vi "GetMetadataCluster.vi"(7 "Message":refnum<class "Message.lvclass">) -> (3 "MetadataCluster":T1 {"AbsoluteTime" format="%<%x %.3X>T"})   [LabVIEW 2020, in "jettl.lvlib" / "Message.lvclass"]
uses:
  Message.lvclass
  LifecycleEnum.ctl
  jettl.lvlib
  TellOriginEnum.ctl
  MetadataCluster.ctl
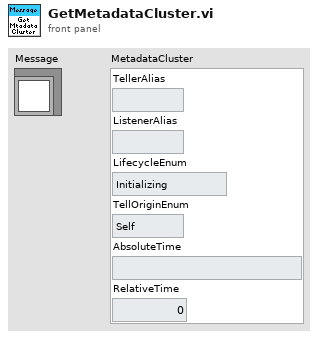
[diagram p1: front panel]
types:
  T1 = typedef "jettl.lvlib/MetadataCluster.ctl" = cluster{"TellerAlias":string, "ListenerAlias":string, "LifecycleEnum":T2, "TellOriginEnum":T3, "AbsoluteTime":timestamp, "RelativeTime":dbl}
  T2 = typedef "jettl.lvlib/LifecycleEnum.ctl" = enum16{"Initializing", "SettingUp", "Starting", "Running", "Stopping", "TearingDown", "Terminated"}
  T3 = typedef "jettl.lvlib/TellOriginEnum.ctl" = enum16{"Self", "Mediator", "Component"}
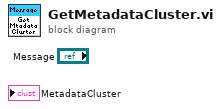
[diagram p0: block diagram]
diagram:
